vi "test2.vi"() -> ()   [LabVIEW 2015]
uses:
  <vilib>/Utility/file.llb/Write Delimited Spreadsheet (DBL).vi
panel:
  in  "mode":string[](array[string])=["off", "on", "mod", "on", "off", "off", "off", "off"]
  in  "am":dbl[](array[numeric])=[0.0, 400.0, 715.0, 340.0, 0.0, 0.0, 0.0, 0.0]
  in  "freq":dbl[](array[numeric])=[0.0, 53.105, 75.715, 67.235, 0.0, 0.0, 0.0, 0.0]
  in  "chnm":i32[](array[numeric])=[1, 2, 3, 4, 5, 6, 7, 8]
  out "- pin":dbl[](array[numeric])=[25.0, 11.0, 22.0, 8.0, 2.0, 16.0, 5.0, 19.0]
  out "+ pin":dbl[](array[numeric])=[12.0, 23.0, 9.0, 20.0, 14.0, 3.0, 17.0, 6.0]
  out "TTL pin":i32[](array[numeric])=[13, 24, 10, 21, 15, 4, 18, 7]
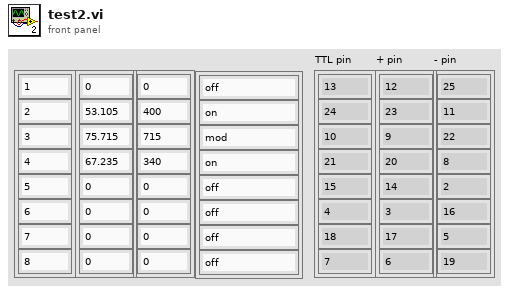
[diagram p1: front panel]
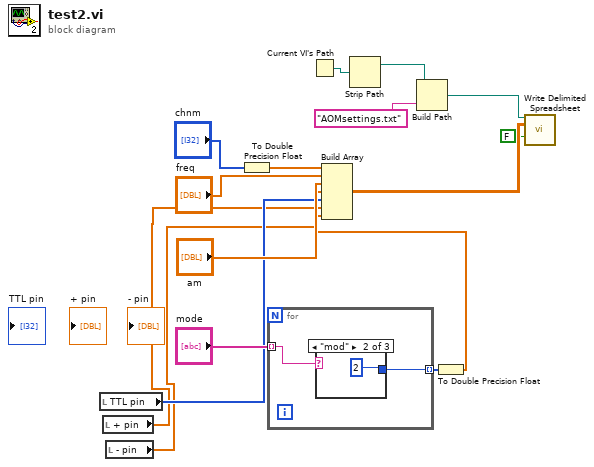
[diagram p0: block diagram]
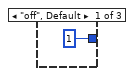
[diagram p2: hidden frame]
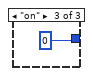
[diagram p3: hidden frame]
diagram:
  n1 = local read "TTL pin"() -> (w3:i32[])
  n2 = local read "+ pin"() -> (w2:dbl[])
  n3 = local read "- pin"() -> (w1:dbl[])
  n4 = To Double Precision Float(number="chnm") -> (double precision float=w11:dbl[])
  n5 = for {
    tunnel: "mode" -> [w18] mode=indexing
    tunnel: [w17] -> w12 mode=indexing
    n6 = case shown="\"mod\"" w18 {
      tunnel: [1 2 0] -> w17
      frame "off", Default {
      }
      frame "mod" {
      }
      frame "on" {
      }
    }
  }
  n7 = Current VI's Path() -> (path=w9:path)
  n8 = Strip Path(path=w9) -> (stripped path=w8:path)  [unwired: 1 out]
  n9 = Build Path(base path=w8, name or relative path="AOMsettings.txt") -> (appended path=w6:path)
  n10 = To Double Precision Float(number=w12) -> (double precision float=w10:dbl[])
  n11 = Build Array(w11, "freq", "am", w10, w3, w2, w1) -> (w5:dbl[][])
  n12 = call-poly <vilib>:"Write Delimited Spreadsheet.vi"("file path (dialog if empty)"=w6, "2D data"=w5, "append to file? (F)"=FALSE) -> ()  [unwired: 11 in, 2 out]
